vi "replaceQueryTokens.vi"(8 "error in (no error)":errorcluster, 10 "Query In":string, 11 "CreditTransaction in":refnum<class "CreditTransaction.lvclass">) -> (0 "error out":errorcluster, 2 "Query Out":string, 3 "CreditTransaction out":refnum<class "CreditTransaction.lvclass">)   [LabVIEW 2020, in "CreditTransaction.lvclass"]
uses:
  CreditTransaction.lvclass
  Transaction/Transaction.lvclass
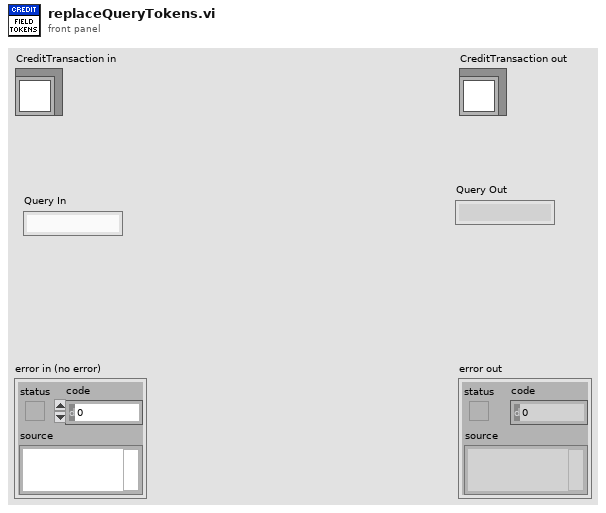
[diagram p1: front panel]
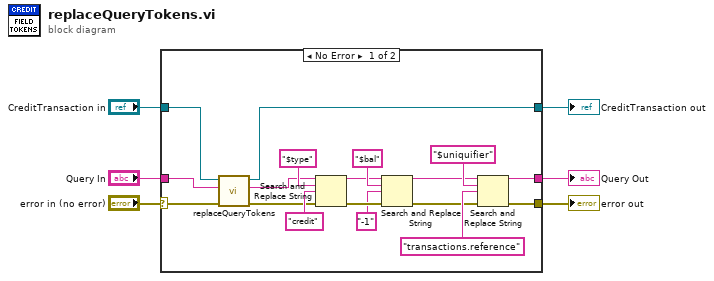
[diagram p0: block diagram]
diagram:
  n1 = case shown="No Error" "error in (no error)" {
    selector: "error in (no error)" -> [w14 w26]
    tunnel: [w24 w27] -> w1
    tunnel: "Query In" -> [w23 w25]
    tunnel: "CreditTransaction in" -> [w17 w27]
    tunnel: [w7 w26] -> w5
    tunnel: [w8 w25] -> w4
    frame No Error {
      n2 = call-parent "replaceQueryTokens.vi"("error in (no error)"=w14, "Query In"=w23, "Transaction in"=w17) -> ("error out"=w19:errorcluster, "Query Out"=w20:string, "Transaction out"=w24:refnum<class "CreditTransaction.lvclass">)  [unwired: 6 in]
      n3 = Search and Replace String(input string=w20, search string="$type", replace string="credit" ("replace string (\"\")"), error in=w19) -> (result string=w16:string, error out=w15:errorcluster)  [unwired: 4 in, 2 out]
      n4 = Search and Replace String(input string=w16, search string="$bal", replace string="-1" ("replace string (\"\")"), error in=w15) -> (result string=w9:string, error out=w10:errorcluster)  [unwired: 4 in, 2 out]
      n5 = Search and Replace String(input string=w9, search string="$uniquifier", replace string="transactions.reference", error in=w10) -> (result string=w8:string, error out=w7:errorcluster)  [unwired: 4 in, 2 out]
    }
    frame Error {
    }
  }
  "error out" <- w5
  "CreditTransaction out" <- w1
  "Query Out" <- w4
